vi "Vision Processing.vi"(8 "error in (no error)":errorcluster, 11 "Image Size":T1=enum."320x240") -> ()   [LabVIEW 2023]
uses:
  <vilib>/Rock Robotics/WPI/Camera/WPI_CameraImageSize.ctl
  <vilib>/Rock Robotics/WPI/Camera/WPI_CameraWhite Balance Values.ctl
  <vilib>/Rock Robotics/WPI/Camera/WPI_CameraExposure Values.ctl
  <vilib>/Rock Robotics/WPI/Camera/WPI_CameraFrameRate.ctl
  Framework/Robot Global Data.vi
  <vilib>/Rock Robotics/Network Tables/NT Write Number.vi
  Vision Support Code/Camera Types.ctl
panel:
  out "loop ms":u32
  out "Instructions:":string="Connect a USB or IP camera to your roboRIO. If using a ring light and retroreflective tape, use Camera Settings outside the loop create a dark image with bright and colorful stripes. If used wihtout a ring light, brighten the images so that stripes are visible.\n\nLED Color can encoded as HSL or related color modes. Calibrate to the same color as the strips being reflected to the camera. Unlike the desktop example, this LED color must be set by hand. You can also put the calibration on the dashboard and send the LED Color to the RT code using Network Tables.\n\nThe Display buttons affects whether images are displayed on the panel. It takes quite a bit of CPU  to compress and transmit the images for display.\n\nAdjust Score Cutoff to make the code more or less picky. If the color is not very unique, you may need to increase the number of particles considered. The diagram uses a Size Limit to ignore colored things that are too small. You may need to adjust it if you are targetting from far away.\n\nResults give you the distance to the target, the center and box in a normalized (-1 to 1) and pixel coordinates.\n\nBe sure to read about setting camera exposure and brightness to help simplify your image and acquire color saturated images.\n\nThere are lots of comments on the diagram to explain the code."
  # "Good target, distance ft"
  # "Bad target"
  # "Score in %"
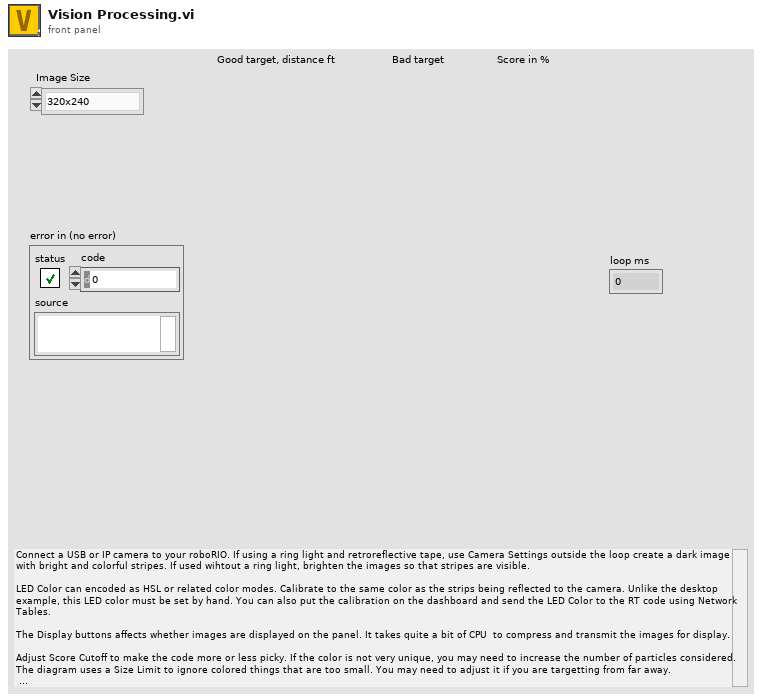
[diagram p1: front panel]
types:
  T1 = typedef "WPI_CameraImageSize.ctl" = enum16{"640x480", "320x240", "160x120", "Custom"}
  T2 = typedef "WPI_CameraFrameRate.ctl" = u32
  T3 = typedef "WPI_CameraExposure Values.ctl" = enum16{"Auto", "Flicker-free 50 Hz", "Flicker-free 60 Hz", "Hold current", "Custom"}
  T4 = typedef "WPI_CameraWhite Balance Values.ctl" = enum16{"Auto", "Fixed indoor", "Fixed outdoor 1", "Fixed outdoor 2", "Fixed fluorescent 1", "Fixed fluorescent 2", "Hold current", "Custom"}
  T5 = typedef "Image Type" = u32
  T6 = typedef "WPI_CameraDevRef.ctl" = cluster{"Camera Address":string, "CameraStatus":errorcluster}
  T7 = typedef "IMAQ Image.ctl" = refnum<image>
  T8 = typedef "Camera Types.ctl" = enum16{"206", "1011", "1013", "MS HD3000 square", "MS HD3000 640x480"}
  T9 = cluster{"tag ID":i32, "Center":cluster{"X":dbl, "Y":dbl}, "homography matrix":dbl[], "decision margin":dbl, "Hamming Dist":i32, "corner points":cluster{"X":dbl, "Y":dbl}[], "Tag Family":string}[]
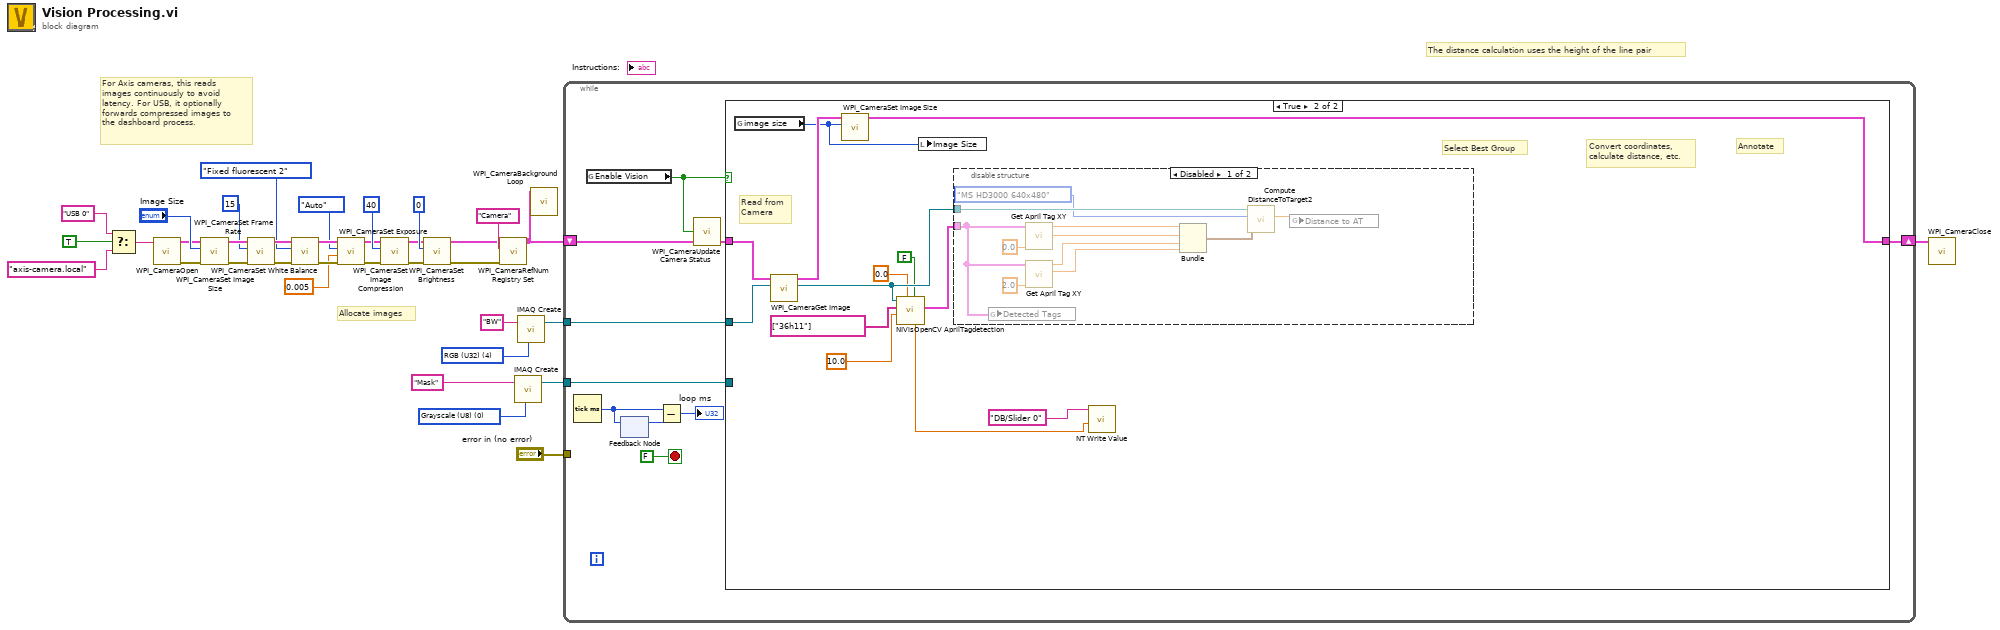
[diagram p0: block diagram]
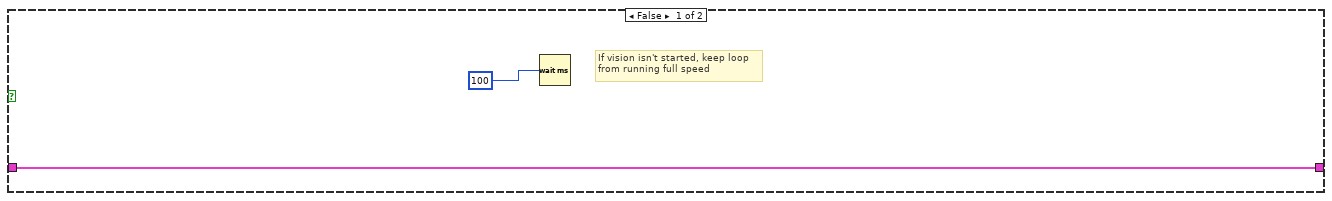
[diagram p2: hidden frame]
diagram:
  w33 = T5 0 items=["Grayscale (U8)", "Grayscale (I16)", "Grayscale (SGL)", "Complex (CSG)", "RGB (U32)", "HSL (U32)", "RGB (U64)", "Grayscale (U16)"] ("Image Type")
  w34 = T5 4 items=["Grayscale (U8)", "Grayscale (I16)", "Grayscale (SGL)", "Complex (CSG)", "RGB (U32)", "HSL (U32)", "RGB (U64)", "Grayscale (U16)"] ("Image Type")
  # "For Axis cameras, this reads\nimages continuously to avoid\nlatency. For USB, it optionally\nforwards compressed images to\nthe dashboard process."
  # "The distance calculation uses the height of the line pair"
  # "Allocate images"
  n1 = Select(t="USB 0" ("format string"), s=TRUE ("dot notation? (F)"), f="axis-camera.local" ("format string")) -> (s? t:f=w7:string)
  n2 = call <vilib>:"WPI_CameraOpen.vi"("Camera Address"=w7) -> ("error out"=w18:errorcluster, "CameraDevRef"=w19:T6)  [unwired: 2 in, 7 out]
  n3 = call <vilib>:"WPI_CameraSet Image Size.vi"("error in (no error)"=w18, "Image Size"="Image Size", "CameraDevRef"=w19) -> ("error out"=w17:errorcluster, "CameraDevRef Out"=w20:T6)  [unwired: 1 in, 6 out]
  n4 = call <vilib>:"WPI_CameraSet Frame Rate.vi"("error in (no error)"=w17, "Frame Rate (fps)"=T2 15, "CameraDevRef"=w20) -> ("error out"=w16:errorcluster, "CameraDevRef Out"=w22:T6)  [unwired: 7 out]
  n5 = call <vilib>:"WPI_CameraSet White Balance.vi"("error in (no error)"=w16, "White Balance"=WPI_CameraWhite_Balance_Values."Fixed fluorescent 2", "CameraDevRef"=w22) -> ("error out"=w15:errorcluster, "CameraDevRef Out"=w21:T6)  [unwired: 1 in, 6 out]
  n6 = call <vilib>:"WPI_CameraSet Exposure.vi"("error in (no error)"=w15, "Exposure (%)"=0.005, "Exposure"=WPI_CameraExposure_Values."Auto", "CameraDevRef"=w21) -> ("error out"=w14:errorcluster, "CameraDevRef Out"=w24:T6)  [unwired: 6 out]
  n7 = call <vilib>:"WPI_CameraSet Image Compression.vi"("error in (no error)"=w14, "Compression"=40, "CameraDevRef"=w24) -> ("error out"=w13:errorcluster, "CameraDevRef Out"=w23:T6)  [unwired: 7 out]
  n8 = call <vilib>:"WPI_CameraSet Brightness.vi"("error in (no error)"=w13, "Brightness"=0, "CameraDevRef"=w23) -> ("error out"=w1:errorcluster, "CameraDevRef Out"=w2:T6)  [unwired: 1 in, 6 out]
  n9 = call <vilib>:"WPI_CameraRefNum Registry Set.vi"("error in (no error)"=w1, "refnum name"="Camera", "CameraDevRef"=w2) -> ("CameraDevRef"=w6:T6)  [unwired: 1 in, 7 out]
  n10 = call "IMAQ Create"("Image Name"="Mask", "Image Type"=w33) -> ("New Image"=w31:T7)  [unwired: 2 in, 2 out]
  n11 = call "IMAQ Create"("Image Name"="BW", "Image Type"=w34) -> ("New Image"=w30:T7)  [unwired: 2 in, 2 out]
  n12 = call <vilib>:"WPI_CameraBackground Loop.vi"("CameraDevRef"=w6) -> ()  [unwired: 11 in]
  n13 = while {
    tunnel: w30 -> [w43]
    tunnel: w31 -> [w44]
    shift-right: [w42] -> w5
    shift-left: w6 -> [w41]
    tunnel: "error in (no error)" -> [_]
    stop <- FALSE stop-if-true
    n14 = Tick Count (ms)() -> (millisecond timer value=w37:u32)
    n15 = global read "Robot Global Data.vi" "Enable Vision"() -> (w39:bool)
    n16 = feedback-in #1(w37) -> ()
    n17 = feedback #1() -> (w38:u32)  [unwired: 1 in]
    n18 = Subtract(x=w37, y=w38) -> (x-y=→"loop ms":u32)
    n19 = call <vilib>:"WPI_CameraUpdate Camera Status.vi"("CameraDevRef In"=w41, "Enable Vision"=w39) -> ("CameraDevRef Out"=w40:T6)  [unwired: 3 in]
    n20 = case shown="True" w39 {
      tunnel: w44 -> [_ _]
      tunnel: w40 -> [w47 w60]
      tunnel: w43 -> [_ w59]
      tunnel: [w47 w57] -> w42
      frame False {
        # "If vision isn't started, keep loop\nfrom running full speed"
        n21 = Wait (ms)(milliseconds to wait=u32 100) -> ()  [unwired: 1 out]
      }
      frame True {
        # "Read from\nCamera"
        # "Convert coordinates,\ncalculate distance, etc."
        # "Annotate"
        # "Select Best Group"
        n22 = global read "Robot Global Data.vi" "image size"() -> (w56:T1)
        n23 = call <vilib>:"WPI_CameraGet Image.vi"("Image"=w59, "CameraDevRef"=w60) -> ("Image Out"=w55:T7, "CameraDevRef Out"=w58:T6)  [unwired: 7 in, 1 out]
        n24 = call <vilib>:"WPI_CameraSet Image Size.vi"("Image Size"=w56, "CameraDevRef"=w58) -> ("CameraDevRef Out"=w57:T6)  [unwired: 2 in, 7 out]
        n25 = call <vilib>:"NIVisOpenCV AprilTagdetection.vi"("refine Edges"=FALSE, "blur"=0.0, "decimate"=10.0, "Tag Familys"=string[] ["36h11"], "Image Src"=w55) -> ("Detected Tags"=w53:T9, "exec time (s)"=w51:dbl)  [unwired: 3 in, 2 out]
        n26 = local write "Image Size"(w56) -> ()
        n27 = disable-structure shown="Disabled" {
          disable-tunnel: w55 -> [w71 _]
          disable-tunnel: w53 -> [w61 _]
          frame Disabled {
            n28 = global write "Robot Global Data.vi" "Detected Tags"(w61) -> ()
            n29 = call "Get April Tag XY.vi"("Corner"=0.0, "Detected Tags"=w61) -> ("Y"=w66:dbl, "X"=w67:dbl)  [unwired: 7 in]
            n30 = call "Get April Tag XY.vi"("Corner"=2.0, "Detected Tags"=w61) -> ("Y"=w63:dbl, "X"=w64:dbl)  [unwired: 7 in]
            n31 = Bundle("X"=w67, "Y"=w66, "X"=w64, "Y"=w63) -> (w68:cluster{"X":dbl, "Y":dbl, "X":dbl, "Y":dbl})  [unwired: 1 in]
            n32 = call "Compute DistanceToTarget2.vi"("Rect"=w68, "Camera Type"=Camera_Types."MS HD3000 640x480", "Image Src"=w71) -> ("Distance (ft)"=w62:dbl)  [unwired: 7 in, 1 out]
            n33 = global write "Robot Global Data.vi" "Distance to AT"(w62) -> ()
          }
          frame Enabled {
          }
        }
        n34 = call-poly <vilib>:"NT Write Value.vi"("value"=w51, "name"="DB/Slider 0") -> ()  [unwired: 9 in, 1 out]
      }
    }
  }
  n35 = call <vilib>:"WPI_CameraClose.vi"("CameraDevRef"=w5) -> ()  [unwired: 1 in, 10 out]
